vi "TemperatureGradientTest.vi"(10 "Temp Out":dbl[](array[numeric]), 11 "mean":dbl) -> (2 "Gradient":dbl, 3 "Gradient?":bool)   [LabVIEW 2018, in "Analysis.lvlib"]
doc: "This VI compares the average cal-tube temperature in degrees C to the average temperature of the sounding tube. If the absolute value of the difference is greater than the threshold, the boolean indicator returns FALSE."
uses:
  Analysis.lvlib
  <vilib>/Analysis/baseanly.llb/Mean (DBL).vi
  <vilib>/Analysis/NI_AALBase.lvlib
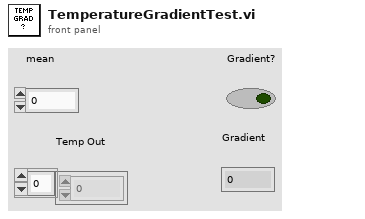
[diagram p1: front panel]
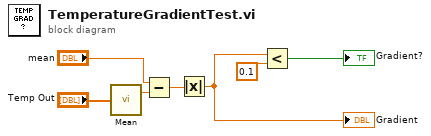
[diagram p0: block diagram]
diagram:
  n1 = call-poly <vilib>:"Mean.vi"("X"="Temp Out") -> ("mean"=w1:dbl)  [unwired: 1 out]
  n2 = Subtract(x="mean", y=w1) -> (x-y=w2:dbl)
  n3 = Absolute Value(x=w2) -> (abs(x)=w5:dbl)
  "Gradient" <- w5
  n4 = Less?(x=w5, y=0.1) -> (x < y?=→"Gradient?":bool)
